vi "Stop.vi"(8 "error in":errorcluster, 11 "Red-y Read Write CFG in":refnum<class "Red-y Read Write CFG.lvclass">) -> (0 "error out":errorcluster, 3 "Red-y Read Write CFG out":refnum<class "Red-y Read Write CFG.lvclass">)   [LabVIEW 2023, in "Red-y Read Write CFG.lvclass"]
uses:
  Red-y Read Write CFG.lvclass
  Red-y Read Write CFG.lvclass/Red-y Read Write CFG.ctl
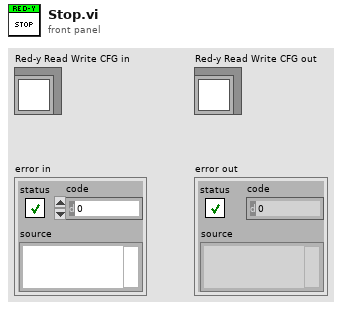
[diagram p1: front panel]
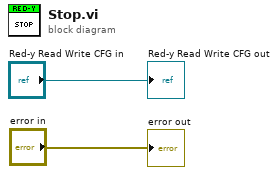
[diagram p0: block diagram]
diagram:
  "error out" <- "error in"
  "Red-y Read Write CFG out" <- "Red-y Read Write CFG in"
